vi "Write channel config.vi"(8 "error in (no error)":errorcluster, 10 "channel config":T1, 11 "Class 2 in":refnum<class "Class 2.lvclass">) -> (0 "error out":errorcluster, 3 "Class 2 out":refnum<class "Class 2.lvclass">)   [LabVIEW 2016, in "Data Sharing Framework.Runtime.lvlib" / "Class 2.lvclass"]
uses:
  Class 2.lvclass
  Typedefs/Channel Configuration.ctl
  <vilib>/NI Veristand/VeriStand Data/Typedefs/Typedefs.Data Types.ctl
  Class 2.lvclass/Class 2.ctl
  <vilib>/NI Veristand/VeriStand Data/VeriStand Data.lvlib
  Classes/Configuration.Channel/Configuration.Channel.lvclass
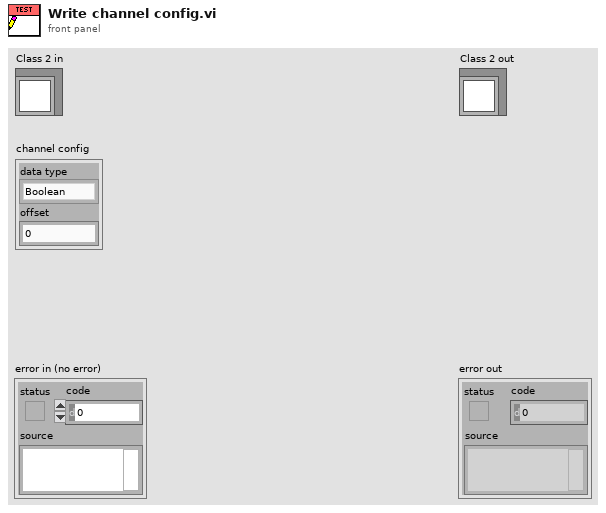
[diagram p1: front panel]
types:
  T1 = typedef "Data Sharing Framework.Configuration.lvlib/Configuration.Channel.lvclass/Channel Configuration.ctl" = cluster{"data type":T2, "offset":u64}
  T2 = typedef "VeriStand Data.lvlib/Typedefs.Data Types.ctl" = enum16{"Boolean", "Single", "Double", "I8", "I16", "I32", "I64", "U8", "U16", "U32", "U64"}
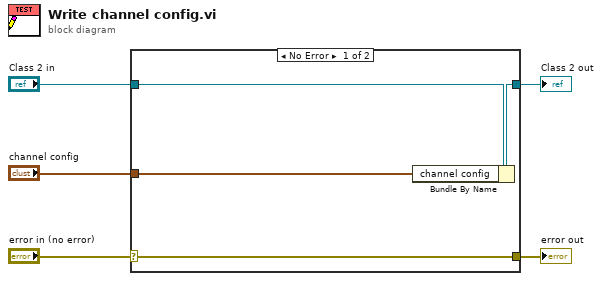
[diagram p0: block diagram]
diagram:
  n1 = case shown="No Error" "error in (no error)" {
    selector: "error in (no error)" -> [w9 w10]
    tunnel: [w9 w10] -> w4
    tunnel: [w7 w11] -> w2
    tunnel: "Class 2 in" -> [w8 w11]
    tunnel: "channel config" -> [w6 _]
    frame No Error {
      n2 = Bundle By Name(cluster=w8, "channel config"=w6) -> (w7:refnum<class "Class 2.lvclass">)
    }
    frame Error {
    }
  }
  "error out" <- w4
  "Class 2 out" <- w2
